vi "Read Current Leakage.vi"(0 "VISA resource name":refnum<visa-resource-name>, 1 "Source Current Limit (1 A)":dbl=1.0, 2 "Source Delay (0.3 S)":dbl=0.3, 5 "Source Measure Unit Channel (0: Channel A)":i32(ring) items=["Channel A", "Channel B"], 7 "Voltage Level (0 V)":dbl, 11 "error in (no error)":errorcluster, 12 "Measure Current Limit (1E-5 A)":dbl=1e-05, 13 "Measure Delay (0.1 S)":dbl=0.1) -> (4 "VISA resource name out":refnum<visa-resource-name>, 6 "Leakage Current":dbl, 15 "error out":errorcluster)   [LabVIEW 2019, in "Keithley 2600 Series.lvlib"]
doc: "Performs a current leakage measurement after stepping the output voltage."
uses:
  Keithley 2600 Series.lvlib
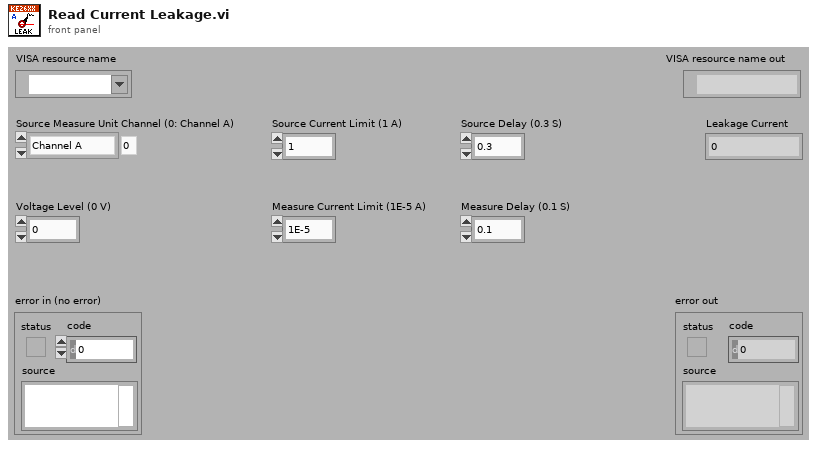
[diagram p1: front panel]
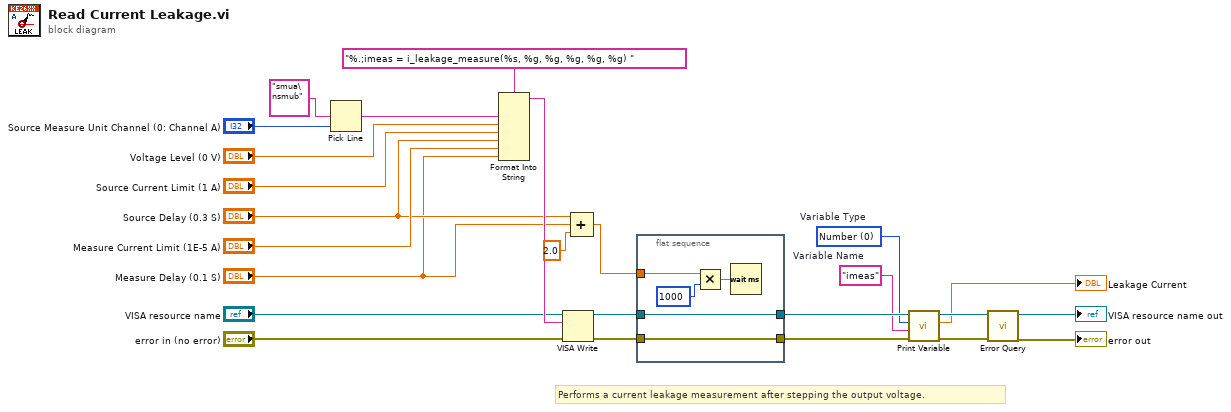
[diagram p0: block diagram]
diagram:
  w2 = "imeas"  # Variable Name
  w3 = 0 items=["Number", "Message"]  # Variable Type
  # "Performs a current leakage measurement after stepping the output voltage."
  n1 = Pick Line(multi-line string="smua\nsmub", line index="Source Measure Unit Channel (0: Channel A)") -> (output string=w14:string)  [unwired: 1 in]
  n2 = Format Into String(format string="%.;imeas = i_leakage_measure(%s, %g, %g, %g, %g, %g) ", w14, "Voltage Level (0 V)", "Source Current Limit (1 A)", "Source Delay (0.3 S)", "Measure Current Limit (1E-5 A)", "Measure Delay (0.1 S)") -> (resulting string=w21:string)  [unwired: 2 in, 1 out]
  n3 = VISA Write(VISA resource name="VISA resource name", write buffer=w21, error in (no error)="error in (no error)") -> (VISA resource name out=w13:refnum<visa-resource-name>, error out=w12:errorcluster)  [unwired: 1 out]
  n4 = Compound Arithmetic op=ADD("Source Delay (0.3 S)", "Measure Delay (0.1 S)", 2.0 ("value")) -> (w9:dbl)
  n5 = flat-sequence {
    tunnel: w13 -> [w30]
    tunnel: w12 -> [w29]
    tunnel: [w30] -> w7
    tunnel: [w29] -> w5
    tunnel: w9 -> [w26]
    frame #0 {
      n6 = Multiply(x=w26, y=1000) -> (x*y=w28:dbl)
      n7 = Wait (ms)(milliseconds to wait=w28) -> ()  [unwired: 1 out]
    }
  }
  n8 = call "Print Variable.vi"("error in (no error)"=w5, "Variable Name"=w2, "Variable Type (0: Number)"=w3, "VISA resource name"=w7) -> ("error out"=w4:errorcluster, "Number"=→"Leakage Current":dbl, "VISA resource name out"=w6:refnum<visa-resource-name>)  [unwired: 4 in, 1 out]
  n9 = call "Error Query.vi"("error in (no error)"=w4, "VISA resource name"=w6) -> ("error out"=→"error out":errorcluster, "VISA resource name out"=→"VISA resource name out":refnum<visa-resource-name>)  [unwired: 6 in, 2 out]
